vi "fan.vi"   [LabVIEW 2020]
uses:
  <vilib>/sound2/lvsound2.llb/Sound File Read Open.vi
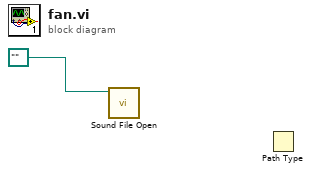
[diagram p0: block diagram]
diagram:
  n1 = call-poly <vilib>:"Sound File Open.vi"("path"=path "") -> ()  [unwired: 9 in, 2 out]
  n2 = Path Type() -> ()  [unwired: 1 in, 1 out]
